vi "parse response value.vi"(11 "Element":u32) -> (0 "data":u8, 1 "index":u8, 2 "device":u8, 3 "header":T1=enum."Input")   [LabVIEW 2013, in "dynamic profibus.lvlib"]
uses:
  dynamic profibus.lvlib
  profibus master transmit header.ctl
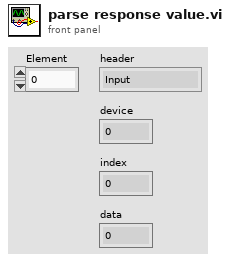
[diagram p1: front panel]
types:
  T1 = typedef "dynamic profibus.lvlib/profibus master transmit header.ctl" = enum8{"Error", "Input", "Diagnostic", "input size", "output size"}
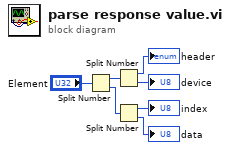
[diagram p0: block diagram]
diagram:
  n1 = Split Number(x="Element") -> (hi(x)=w7:u16, lo(x)=w6:u16)
  n2 = Split Number(x=w7) -> (hi(x)=→"header":u8, lo(x)=→"device":u8)
  n3 = Split Number(x=w6) -> (hi(x)=→"index":u8, lo(x)=→"data":u8)
